vi "cw_5_4.vi"() -> ()   [LabVIEW 2022 SP3]
panel:
  in  "OK Button":bool
  in  "stop":bool
  in  "User":string
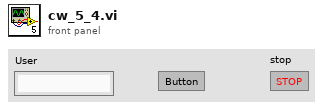
[diagram p1: front panel]
types:
  T1 = enum16{"open", "replace", "create", "open or create", "replace or create", "replace or create with confirmation"}
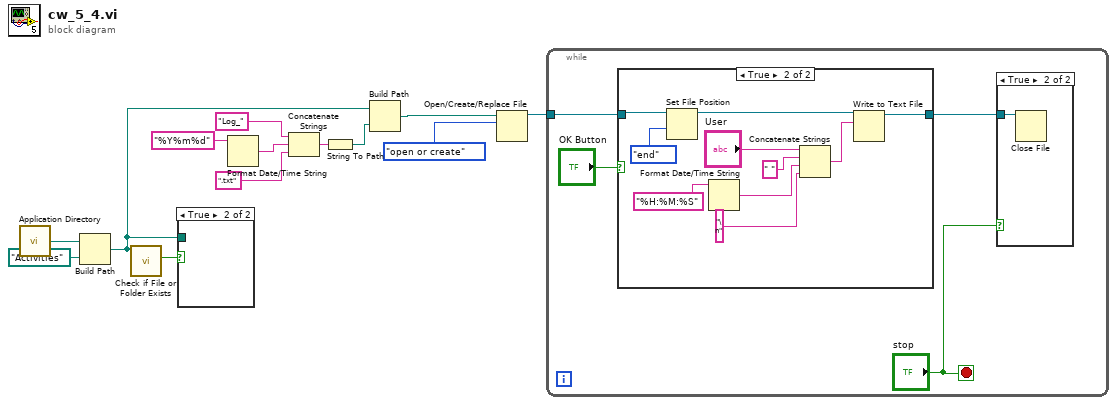
[diagram p0: block diagram]
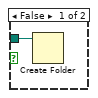
[diagram p4: hidden frame]
diagram:
  n1 = call <vilib>:"Application Directory.vi"() -> ("Application Directory"=w13:path)
  n2 = Build Path(base path=w13, name or relative path=path "Activities") -> (appended path=w10:path)
  n3 = call <vilib>:"Check if File or Folder Exists.vi"("path"=w10) -> ("file or folder exists?"=w11:bool)  [unwired: 8 in, 2 out]
  n4 = case shown="True" w11 {
    tunnel: w10 -> [w14 _]
    frame False {
      n5 = Create Folder(path (use dialog)=w14) -> ()  [unwired: 2 in, 3 out]
    }
    frame True {
    }
  }
  n6 = Format Date/Time String(time format string (%c)="%Y%m%d") -> (date/time string=w3:string)  [unwired: 2 in]
  n7 = Concatenate Strings("Log_" ("string"), w3, ".txt" ("string")) -> (w9:string)
  n8 = String To Path(string=w9) -> (path=w8:path)
  n9 = Build Path(base path=w10, name or relative path=w8) -> (appended path=w4:path)
  n10 = Open/Create/Replace File(file path (use dialog)=w4, operation (0:open)=T1."open or create") -> (refnum out=w1:refnum<file>)  [unwired: 4 in, 2 out]
  n11 = while {
    tunnel: w1 -> [w15]
    stop <- "stop" stop-if-true
    n12 = case shown="True" "OK Button" {
      tunnel: [w20 w28] -> w16
      tunnel: w15 -> [w20 w23]
      frame False {
      }
      frame True {
        n13 = Set File Position(refnum=w23, from (0:start)=enum16{"start", "end", "current"}."end") -> (refnum out=w22:refnum<file>)  [unwired: 2 in, 1 out]
        n14 = Format Date/Time String(time format string (%c)="%H:%M:%S") -> (date/time string=w25:string)  [unwired: 2 in]
        n15 = Concatenate Strings("User", " " ("string"), w25, "\n" ("string")) -> (w29:string)
        n16 = Write to Text File(file (use dialog)=w22, text=w29) -> (refnum out=w28:refnum<file>)  [unwired: 2 in, 2 out]
      }
    }
    n17 = case shown="True" "stop" {
      tunnel: w16 -> [_ w19]
      frame False {
      }
      frame True {
        n18 = Close File(refnum=w19) -> ()  [unwired: 1 in, 2 out]
      }
    }
  }
